vi "hmac_str.vi"(0 "Method":string, 5 "Nonce":string, 7 "Date":string, 9 "ctype":string, 11 "path":string, 12 "query":string) -> (4 "hmac_str":string)   [LabVIEW 2019]
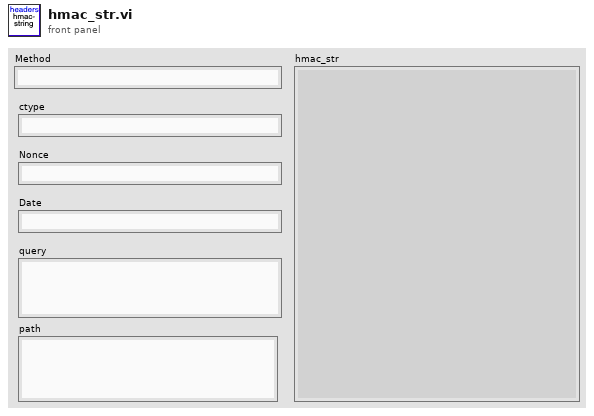
[diagram p1: front panel]
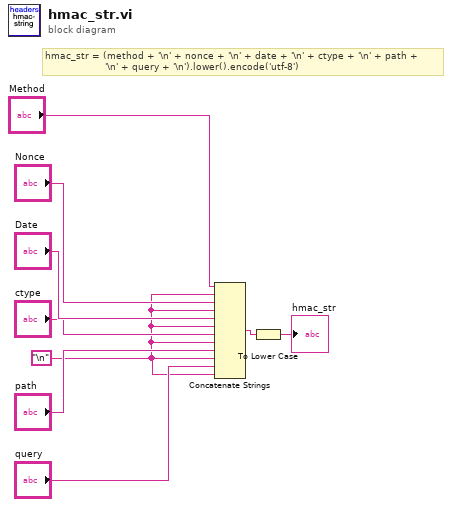
[diagram p0: block diagram]
diagram:
  w1 = "\n"
  # "hmac_str = (method + '\\n' + nonce + '\\n' + date + '\\n' + ctype + '\\n' + path +\n                    '\\n' + query + '\\n').lower().encode('utf-8')"
  n1 = Concatenate Strings("Method", w1, "Nonce", w1, "Date", w1, "ctype", w1, "path", w1, "query", w1) -> (w4:string)
  n2 = To Lower Case(string=w4) -> (all lower case string=→"hmac_str":string)
